vi "DialogSetIpAddess.vi"(8 "error in (no error)":errorcluster) -> (0 "error out":errorcluster, 2 "Network":string, 3 "NetAddress":u32)   [LabVIEW 2024]
doc: "Use this template to create a dialog box with event handling."
panel:
  in  "Subnet":string
  in  "Available Subnets":i32(listbox)
  in  "OK":bool
  # "Select Subnet"
  # "Input"
  # "Output"
  # "Local"
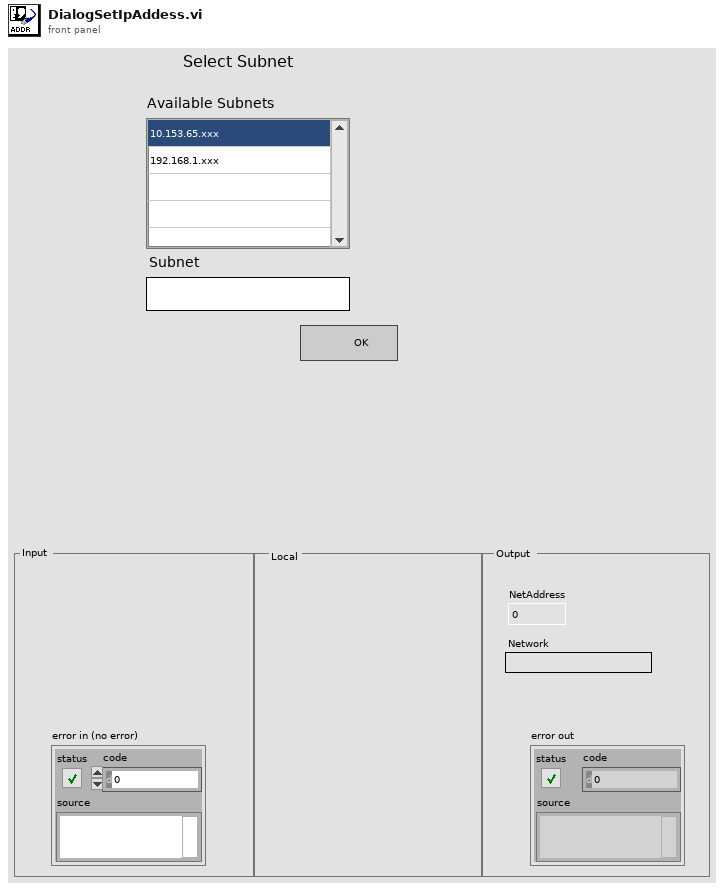
[diagram p1: front panel]
types:
  T1 = enum8{"Enabled", "Disabled", "Disabled and Grayed Out"}
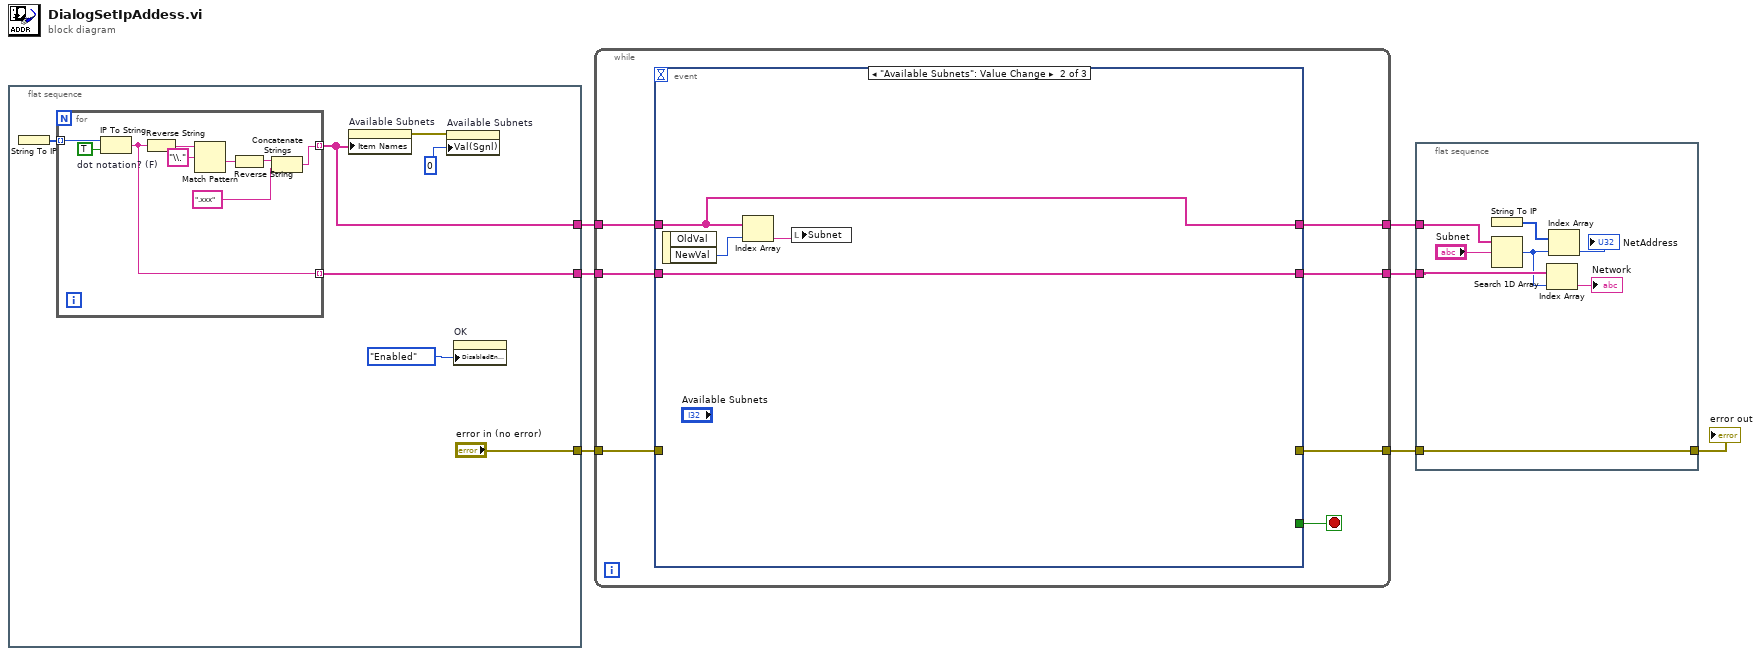
[diagram p0: block diagram]
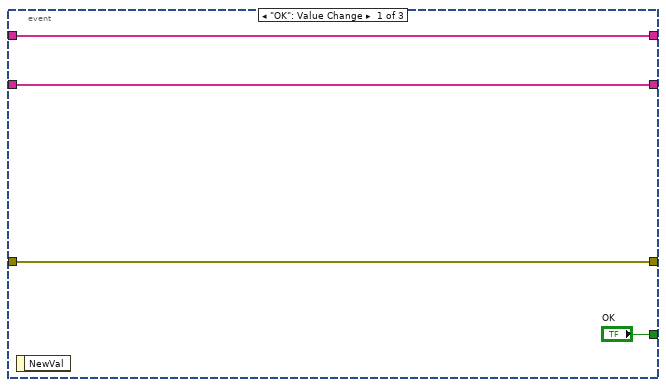
[diagram p2: hidden frame]
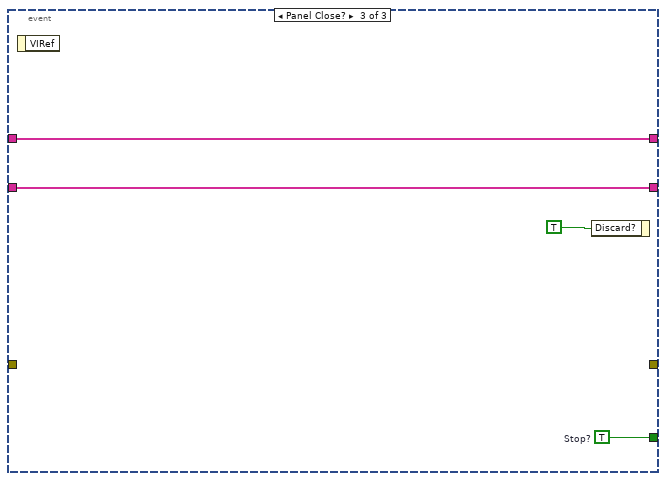
[diagram p3: hidden frame]
diagram:
  n1 = flat-sequence {
    tunnel: ["error in (no error)"] -> w7
    tunnel: [w11] -> w6
    tunnel: [w8] -> w3
    frame #0 {
      n2 = String To IP() -> (0:w12:u32[])  [unwired: 1 in]
      n3 = for {
        tunnel: w12 -> [w23] mode=indexing
        tunnel: [w16] -> w11 mode=indexing
        tunnel: [w15] -> w8 mode=indexing
        w22 = TRUE  # dot notation? (F)
        n4 = IP To String(1:w22, 2:w23) -> (0:w15:string)
        n5 = Reverse String(1:w15) -> (0:w21:string)
        n6 = Match Pattern(string=w21, regular expression="\\.") -> (after substring=w19:string)  [unwired: 1 in, 3 out]
        n7 = Reverse String(1:w19) -> (0:w18:string)
        n8 = Concatenate Strings(w18, ".xxx" ("regular expression")) -> (w16:string)
      }
      n9 = property on="Available Subnets" class="LstBox (strict)"("Item Names"=w11) -> (error out=w10:errorcluster)  [unwired: 2 in, 1 out]
      n10 = property on="Available Subnets" class="LstBox (strict)"(error in=w10, "Val(Sgnl)"=0 ("Value (Signaling)")) -> ()  [unwired: 1 in, 2 out]
      n11 = property on="OK" class="Bool"("DisabledEnum"=T1."Enabled" ("Disabled")) -> ()  [unwired: 2 in, 2 out]
    }
  }
  n12 = while {
    tunnel: w7 -> [w29]
    tunnel: w6 -> [w28]
    tunnel: [w27] -> w5
    tunnel: w3 -> [w26]
    tunnel: [w25] -> w2
    tunnel: [w24] -> w1
    stop <- w30 stop-if-true
    n13 = event shown="[1] \"Available Subnets\": Value Change" {
      selector: _ -> [_ _ _]
      dyn-events: _ -> [_ _ _]
      timeout: _ -> [_ _ _]
      tunnel: ["OK" _ w41] -> w30
      tunnel: w29 -> [w33 _ _]
      tunnel: w28 -> [w32 w35 w40]
      tunnel: [w33 _ _] -> w27
      tunnel: w26 -> [w31 w36 w39]
      tunnel: [w32 w35 w40] -> w25
      tunnel: [w31 w36 w39] -> w24
      event "OK": Value Change {
        n14 = event-data() -> ()  [unwired: 1 in, 1 out]
      }
      event "Available Subnets": Value Change {
        n15 = event-data() -> ("NewVal"=w38:i32)  [unwired: 1 in, 1 out]
        n16 = Index Array(array=w35, index=w38) -> (element=w37:string)
        n17 = local write "Subnet"(w37) -> ()
      }
      event Panel Close? {
        w41 = TRUE  # Stop?
        n18 = event-data() -> ()  [unwired: 1 in, 1 out]
        n19 = event-data("Discard?"=TRUE) -> ()  [unwired: 1 in, 1 out]
      }
    }
  }
  n20 = flat-sequence {
    tunnel: [w50] -> w4
    tunnel: w5 -> [w50]
    tunnel: w2 -> [w49]
    tunnel: w1 -> [w48]
    frame #0 {
      n21 = String To IP() -> (0:w45:u32[])  [unwired: 1 in]
      n22 = Search 1D Array(1D array=w49, element="Subnet") -> (index of element=w44:i32)  [unwired: 1 in]
      n23 = Index Array(array=w48, index=w44) -> (element=→"Network":string)
      n24 = Index Array(array=w45, index=w44) -> (element=→"NetAddress":u32)
    }
  }
  "error out" <- w4
